vi "Configure.vi"(8 "error in (no error)":errorcluster) -> (0 "error out":errorcluster, 1 "valid configuration":bool, 3 "config":T1)   [LabVIEW 2017, in "Trigger.lvlib"]
uses:
  <vilib>/addons/InsightCM/Devices/Shared/Common/Trigger/Trigger.lvlib
  <vilib>/addons/InsightCM/Devices/Shared/Common/Trigger/controls/config.ctl
  <vilib>/addons/PointValueMap/subVIs/Point_Write_double.vi
  <vilib>/addons/InsightCM/Utilities/GlobalConfiguration/GlobalConfiguration.lvlib
  <vilib>/addons/PointValueMap/PointValueMap.lvlib
  <vilib>/addons/InsightCM/Utilities/PropertyHelpers/PropertyHelpers.lvlib
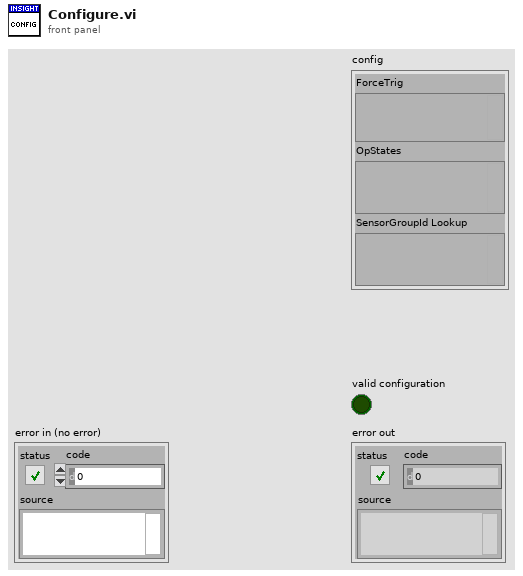
[diagram p1: front panel]
types:
  T1 = typedef "Trigger.lvlib/config.ctl" = cluster{"ForceTrig":variant, "OpStates":variant, "SensorGroupId Lookup":variant}
  T2 = typedef "R2_Device.ctl" = cluster{"Id":string, "Name":string, "DeviceType":string, "HardwareName":string, "IpAddress":string, "HardwareInfo":T3[], "ApplicationType":string, "ApplicationVersion":string, "EquipmentIds":string[], "ConfigurationVersion":string, "State":T4, "Properties":T3[], "DataGroups":T5[], "BurstModeTrigger":T9, "SensorGroups":T10[], "Endpoints":T11[]}
  T3 = typedef "KeyValuePair.ctl" = cluster{"Key":string, "Value":string}
  T4 = typedef "DeviceState.ctl" = cluster{"Disabled":bool}
  T5 = typedef "R2_DataGroup.ctl" = cluster{"Name":string, "OperatingStates":T6[], "Properties":T3[], "EquipmentIds":string[], "AssetNodeId":string}
  T6 = typedef "OperatingState.ctl" = cluster{"Name":string, "Properties":T3[], "Triggers":T7[]}
  T7 = typedef "Trigger.ctl" = cluster{"Type":string, "Expression":string, "Conditions":T8[]}
  T8 = typedef "Condition.ctl" = cluster{"Source":string, "Type":string, "Operator":string, "CompareTo":string, "DwellSeconds":dbl}
  T9 = typedef "BurstModeTrigger.ctl" = cluster{"Trigger":T7, "SampleRate":string, "AcquisitionLength":string}
  T10 = typedef "DeviceSensorGroup.ctl" = cluster{"EquipId":string, "SensorGroupId":string}
  T11 = typedef "WirelessEndpoint.ctl" = cluster{"SerialNumber":string, "Properties":T3[], "Channels":T12[]}
  T12 = typedef "WirelessChannel.ctl" = cluster{"ChannelNumber":i32, "AssetId":string}
  T13 = typedef "MetricDefinitionInstance.ctl" = cluster{"Id":string, "MetricType":string, "Name":string, "Properties":T3[], "HighRate":bool}
  T14 = typedef "SectionKeyValues.ctl" = cluster{"Section":string, "KeyValues":T3[]}
  T15 = typedef "AssetNode.ctl" = cluster{"Id":string, "Type":string, "Name":string, "ParentIds":string[], "State":T16, "MeasType":string, "Properties":T3[], "SensorGroups":T17[], "OperatingStates":T6[], "Metrics":T19[], "TrendAlarmRules":T20[], "References":T23[]}
  T16 = typedef "AssetState.ctl" = cluster{"Disabled":bool}
  T17 = typedef "AssetNodeSensorGroup.ctl" = cluster{"Id":string, "Type":string, "SensorIds":string[], "CollectionConfig":T18, "Properties":T3[]}
  T18 = typedef "WirelessCollectionConfig.ctl" = cluster{"GateCondition":T8, "CronString":string, "RetryIntervalMinutes":string, "MaxRetryAttempts":string}
  T19 = typedef "Metric.ctl" = cluster{"Id":string, "Name":string, "Unit":string, "Properties":T3[], "MetricDefinitionInstanceId":string}
  T20 = typedef "TrendAlarmRule.ctl" = cluster{"Id":string, "AssetNodeId":string, "TrendId":string, "Disabled":bool, "OperatingState":string, "Operator":string, "Hysteresis":dbl, "OnDelaySeconds":dbl, "OffDelaySeconds":dbl, "Levels":T21[], "Properties":T3[]}
  T21 = typedef "TrendAlarmLevel.ctl" = cluster{"Severity":i32, "CompareTo":dbl, "Actions":T22[]}
  T22 = typedef "AlarmAction.ctl" = cluster{"Type":string, "Props":T3[]}
  T23 = typedef "AssetNodeReference.ctl" = cluster{"NodeId":string, "Name":string}
  T24 = typedef "R2_Channel.ctl" = cluster{"Id":string, "DeviceId":string, "Name":string, "ChannelType":string, "HardwareKey":string, "HardwareChannel":string, "DataGroup":string, "Keywords":string[], "EquipmentIds":string[], "Properties":T3[], "Metrics":T19[], "AssetNodeId":string, "MeasType":string, "AssetName":string}
  T25 = typedef "Trigger.lvlib/TriggerOperatingState.ctl" = cluster{"Id":string, "Name":string, "Properties":T3[], "TrendExpression":string, "TrendConditions":T26[], "FileExpression":string, "FileConditions":T26[]}
  T26 = typedef "Trigger.lvlib/TriggerCondition.ctl" = cluster{"Condition":T8, "LatchValue":string, "LatchTime":timestamp}
  T27 = typedef "PointValueMap.lvlib/PointMap.ctl" = refnum<data-value>
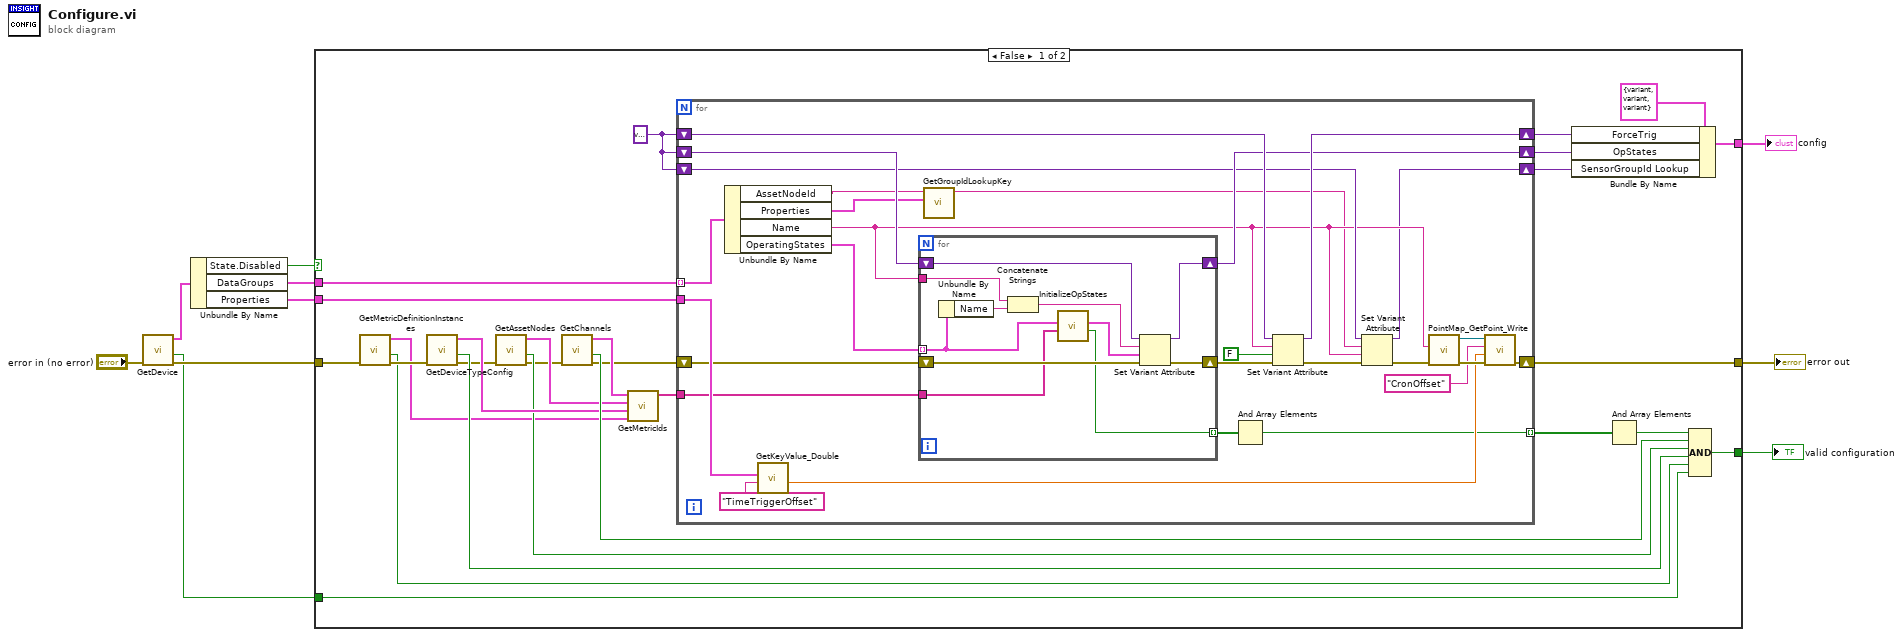
[diagram p0: block diagram]
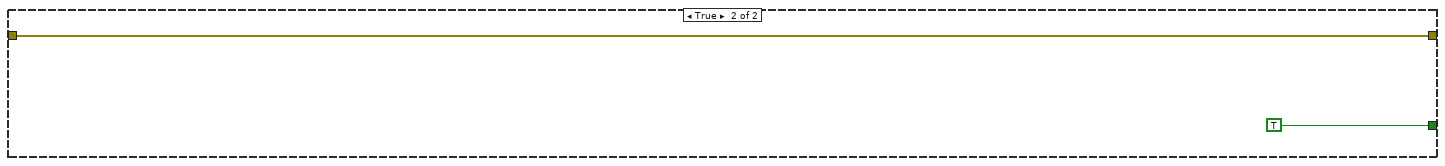
[diagram p2: hidden frame]
diagram:
  n1 = call <vilib>:"GetDevice.vi"("error in (no error)"="error in (no error)") -> ("error out"=w3:errorcluster, "found"=w2:bool, "device configuration"=w9:T2)  [unwired: 8 in]
  n2 = Unbundle By Name(w9) -> ("State.Disabled"=w1:bool, "DataGroups"=w8:T5[], "Properties"=w5:T3[])
  n3 = case shown="False" w1 {
    tunnel: w8 -> [w37 _]
    tunnel: [w36 w77] -> w7
    tunnel: [w32 _] -> w6
    tunnel: w5 -> [w31 _]
    tunnel: [w28 TRUE] -> w4
    tunnel: w3 -> [w17 w77]
    tunnel: w2 -> [w14 _]
    frame False {
      w12 = variant ("Status")
      n4 = call <vilib>:"GetMetricDefinitionInstances.vi"("error in (no error)"=w17) -> ("error out"=w16:errorcluster, "found"=w13:bool, "metrics"=w15:T13[])  [unwired: 8 in]
      n5 = call <vilib>:"GetDeviceTypeConfig.vi"("error in (no error)"=w16) -> ("error out"=w20:errorcluster, "found"=w23:bool, "key values"=w24:T14[])  [unwired: 8 in]
      n6 = call <vilib>:"GetAssetNodes.vi"("error in (no error)"=w20) -> ("error out"=w19:errorcluster, "found"=w22:bool, "AssetNodes"=w21:T15[])  [unwired: 8 in]
      n7 = call <vilib>:"GetChannels.vi"("error in (no error)"=w19) -> ("error out"=w18:errorcluster, "found"=w25:bool, "channels"=w27:T24[])  [unwired: 8 in]
      n8 = call <vilib>:"GetMetricIds.vi"("metrics"=w15, "device type config"=w24, "AssetNodes"=w21, "channels"=w27) -> ("metric ids"=w26:string[])  [unwired: 7 in]
      n9 = for {
        tunnel: w37 -> [w64] mode=indexing
        shift-right: [w62] -> w35
        shift-left: w12 -> [w63]
        shift-right: [w50] -> w34
        shift-left: w12 -> [w51]
        shift-right: [w56] -> w36
        shift-left: w18 -> [w52]
        tunnel: w31 -> [w55]
        tunnel: [w47] -> w30 mode=indexing
        tunnel: w26 -> [w46]
        shift-right: [w41] -> w11
        shift-left: w12 -> [w43]
        n10 = Unbundle By Name(w64) -> ("AssetNodeId"=w39:string, "Properties"=w38:T3[], "Name"=w42:string, "OperatingStates"=w60:T6[])
        n11 = call <vilib>:"GetKeyValue_Double.vi"("key"="TimeTriggerOffset", "key value pairs"=w55) -> ("value"=w53:dbl)  [unwired: 7 in, 2 out]
        n12 = for {
          shift-right: [w72] -> w61
          shift-left: w52 -> [w67]
          tunnel: w60 -> [w73] mode=indexing
          tunnel: w42 -> [w74]
          shift-right: [w71] -> w50
          shift-left: w51 -> [w70]
          tunnel: [w66] -> w48 mode=indexing
          tunnel: w46 -> [w65]
          n13 = Unbundle By Name(w73) -> ("Name"=w75:string)
          n14 = Concatenate Strings(w74, w75) -> (w69:string)
          n15 = call <vilib>:"InitializeOpStates.vi"("metric ids"=w65, "op state in"=w73) -> ("valid config"=w66:bool, "conv op state"=w68:T25)  [unwired: 8 in]
          n16 = Set Variant Attribute(Variant=w70, name=w69, value=w68, error in=w67) -> (Variant out=w71:variant, error out=w72:errorcluster)  [unwired: 1 out]
        }
        n17 = call <vilib>:"GetGroupIdLookupKey.vi"("Properties"=w38, "AssetNodeId"=w39) -> ("group id lookup key"=w40:string)  [unwired: 9 in]
        n18 = And Array Elements(Boolean array=w48) -> (logical AND=w47:bool)
        n19 = Set Variant Attribute(Variant=w63, name=w42, value=FALSE ("ForceTrigger"), error in=w61) -> (Variant out=w62:variant, error out=w45:errorcluster)  [unwired: 1 out]
        n20 = Set Variant Attribute(Variant=w43, name=w40, value=w42, error in=w45) -> (Variant out=w41:variant, error out=w44:errorcluster)  [unwired: 1 out]
        n21 = call <vilib>:"PointMap_Get.vi"("error in (no error)"=w44, "Name"=w42) -> ("error out"=w59:errorcluster, "Map Out"=w58:T27)  [unwired: 7 in, 1 out]
        n22 = call-poly <vilib>:"Point_Write.vi"("Error In"=w59, "Value"=w53, "Tag"="CronOffset", "Map"=w58) -> ("Error Out"=w56:errorcluster)  [unwired: 6 in, 1 out]
      }
      n23 = Bundle By Name(cluster=T1 {"ForceTrig"=variant, "OpStates"=variant, "SensorGroupId Lookup"=variant} ("config"), "ForceTrig"=w35, "OpStates"=w34, "SensorGroupId Lookup"=w11) -> (w32:T1)
      n24 = And Array Elements(Boolean array=w30) -> (logical AND=w29:bool)
      n25 = Compound Arithmetic op=AND(w29, w25, w22, w23, w13, w14) -> (w28:bool)
    }
    frame True {
    }
  }
  "error out" <- w7
  "config" <- w6
  "valid configuration" <- w4
